vi "Dialog Box.vi"(8 "error in (no error)":errorcluster, 11 "Image Gallery in":refnum<class "Image Gallery.lvclass">) -> (0 "error out":errorcluster, 1 "timed out?":bool, 2 "Selection":string, 3 "Image Gallery out":refnum<class "Image Gallery.lvclass">)   [LabVIEW 2012, in "ImageGallery.lvlib" / "Image Gallery.lvclass"]
doc: "This VI contains the code for the dialog box.\nOverride this VI to provide more functionality or to create your own application-specific dialog box."
uses:
  Image Gallery.lvclass
  Fading/_Fade In(I32).vi
  Fading/_Fade Out(I32).vi
panel:
  in  "Close":bool
  in  "Right":bool
  in  "Left":bool
  out "Picture":picture caption="Caption"
  out "String":string
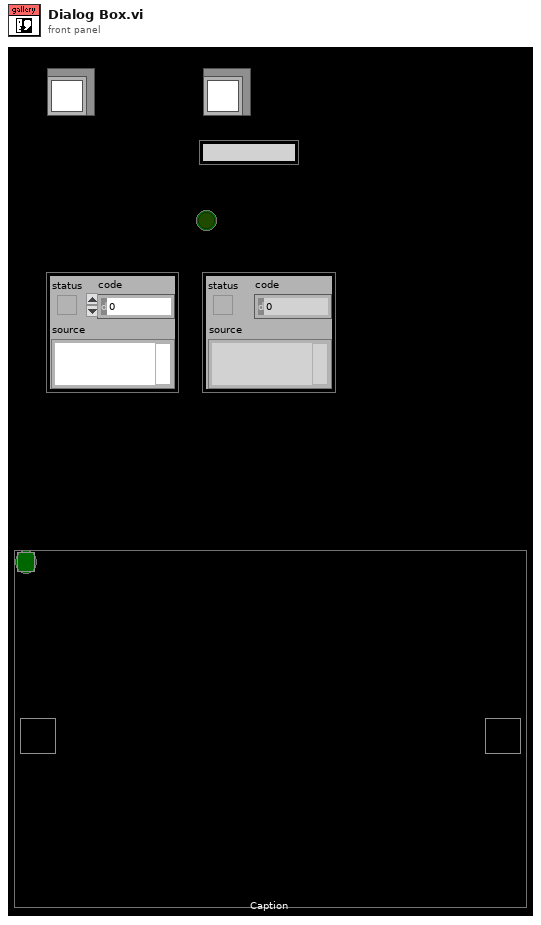
[diagram p1: front panel]
types:
  T1 = cluster{"left":i16, "top":i16, "right":i16, "bottom":i16}
  T2 = typedef "LVPoint32TypeDef.ctl" = cluster{"Horizontal":i32, "Vertical":i32}
  T3 = typedef "LVRectTypeDef.ctl" = cluster{"Left":i16, "Top":i16, "Right":i16, "Bottom":i16}
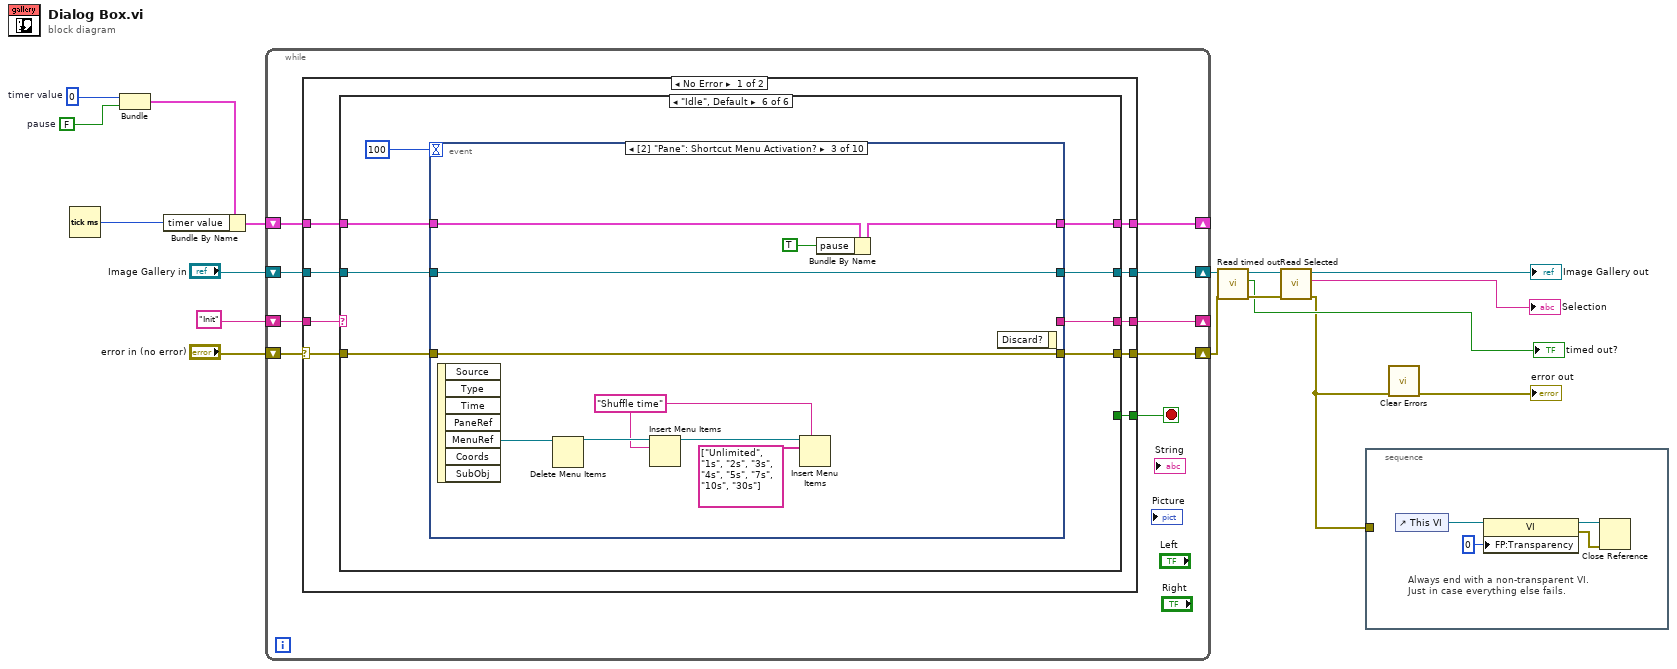
[diagram p0: block diagram]
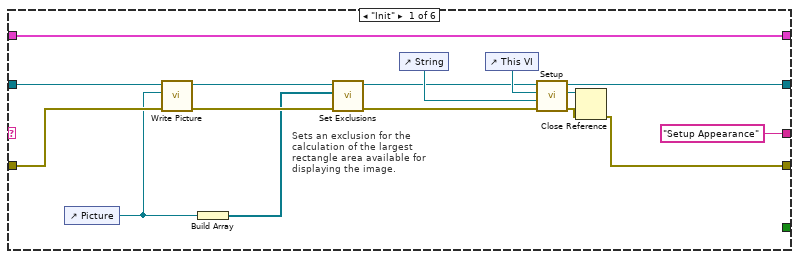
[diagram p2: hidden frame]
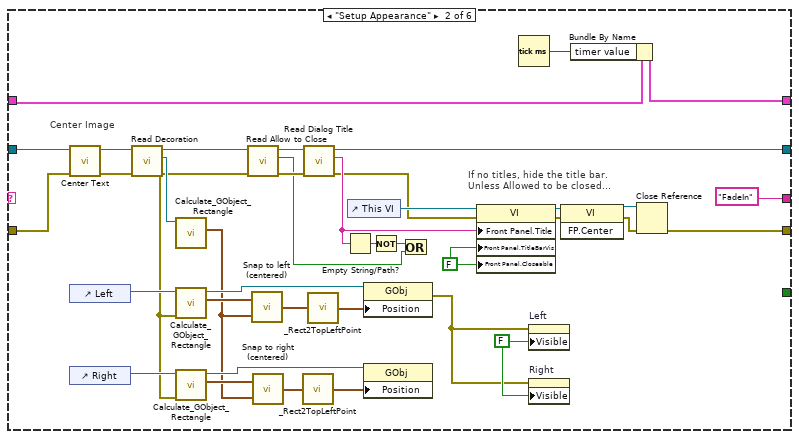
[diagram p3: hidden frame]
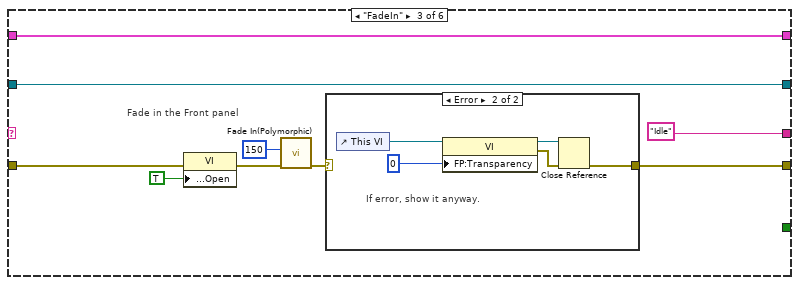
[diagram p4: hidden frame]
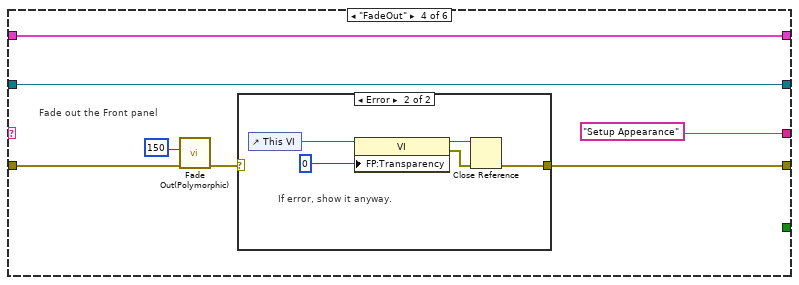
[diagram p6: hidden frame]
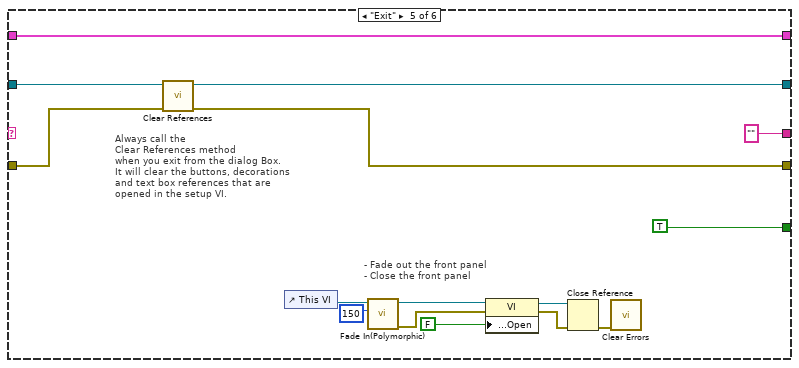
[diagram p8: hidden frame]
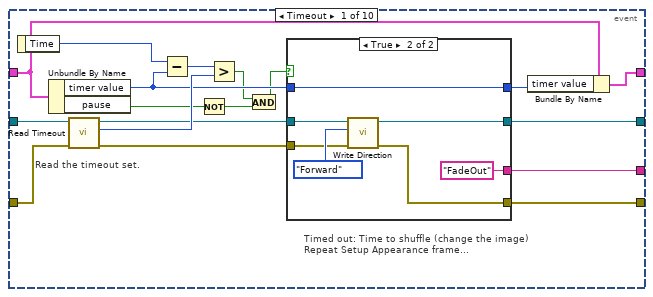
[diagram p9: hidden frame]
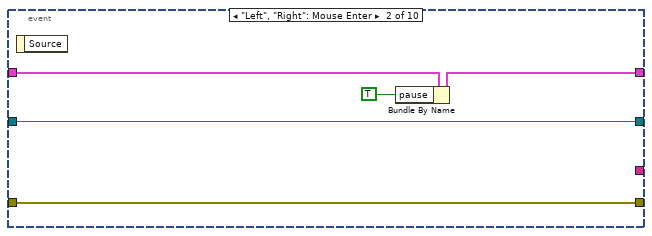
[diagram p11: hidden frame]
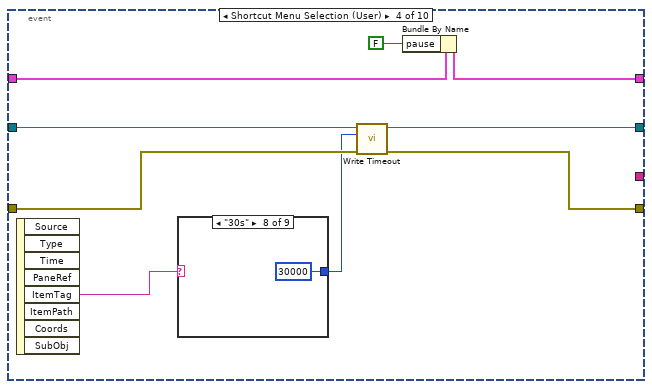
[diagram p12: hidden frame]
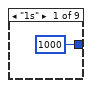
[diagram p13: hidden frame]
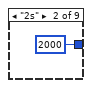
[diagram p14: hidden frame]
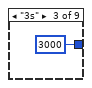
[diagram p15: hidden frame]
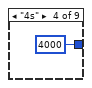
[diagram p16: hidden frame]
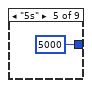
[diagram p17: hidden frame]
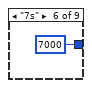
[diagram p18: hidden frame]
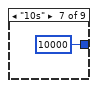
[diagram p19: hidden frame]
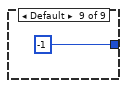
[diagram p20: hidden frame]
diagram:
  w4 = FALSE  # pause
  w5 = u32 0  # timer value
  n1 = Tick Count (ms)() -> (millisecond timer value=w2:u32)
  n2 = Bundle("timer value"=w5, "pause"=w4) -> (w3:cluster{"timer value":u32, "pause":bool})  [unwired: 1 out]
  n3 = Bundle By Name(cluster=w3, "timer value"=w2) -> (w1:cluster{"timer value":u32, "pause":bool})
  n4 = while {
    shift-right: [w22] -> _
    shift-left: "Init" -> [w23]
    shift-right: [w26] -> w16
    shift-left: "Image Gallery in" -> [w25]
    shift-right: [w24] -> w15
    shift-left: "error in (no error)" -> [w20]
    shift-right: [w19] -> _
    shift-left: w1 -> [w18]
    stop <- w21 stop-if-true
    n5 = case shown="No Error" w20 {
      selector: w20 -> [w29 _]
      tunnel: [w35 w250] -> w26
      tunnel: w25 -> [w34 w250]
      tunnel: [w33 errorcluster {"status"=FALSE, "code"=0, "source"=""} ("error out")] -> w24
      tunnel: w23 -> [w32 _]
      tunnel: [w31 "Exit"] -> w22
      tunnel: [w30 _] -> w21
      tunnel: [w28 w247] -> w19
      tunnel: w18 -> [w27 w247]
      frame No Error {
        n6 = case shown="\"Idle\", Default" w32 {
          tunnel: [w49 w81 w99 w112 w123 w141] -> w35
          tunnel: w34 -> [w44 w79 w99 w112 w124 w137]
          tunnel: [w46 w82 w95 w110 w120 w140] -> w33
          tunnel: w29 -> [w43 w78 w94 w107 w122 w136]
          tunnel: ["Setup Appearance" "FadeIn" "Idle" "Setup Appearance" "" w139] -> w31
          tunnel: [_ _ _ _ TRUE _] -> w30
          tunnel: [w36 w52 w91 w106 w119 w134] -> w28
          tunnel: w27 -> [w36 w53 w91 w106 w119 w135]
          frame "Init" {
            # "Sets an exclusion for the\ncalculation of the largest\nrectangle area available for\ndisplaying the image."
            n7 = control-ref of="Picture"() -> (w38:refnum<vi>)
            n8 = call-dynamic "Write Picture.vi"("error in (no error)"=w43, "Picture"=w38, "Image Gallery.lvclass in"=w44) -> ("error out"=w41:errorcluster, "Image Gallery.lvclass out"=w42:refnum<class "Image Gallery.lvclass">)  [unwired: 7 out]
            n9 = Build Array(w38) -> (w37:refnum<vi>[])
            n10 = call-dynamic "Set Exclusions.vi"("error in (no error)"=w41, "Exclusions"=w37, "Dialog in"=w42) -> ("error out"=w39:errorcluster, "Dialog out"=w40:refnum<class "Image Gallery.lvclass">)  [unwired: 7 out]
            n11 = control-ref of="String"() -> (w45:refnum<vi>)
            n12 = control-ref of="This VI"() -> (w50:refnum<vi>)
            n13 = call-dynamic "Setup.vi"("error in (no error)"=w39, "Str Refnum"=w45, "VI Reference"=w50, "Dialog in"=w40) -> ("error out"=w47:errorcluster, "VI reference (dup)"=w48:refnum<vi>, "Dialog out"=w49:refnum<class "Image Gallery.lvclass">)  [unwired: 5 out]
            n14 = Close Reference(reference=w48, error in (no error)=w47) -> (error out=w46:errorcluster)
          }
          frame "Setup Appearance" {
            w56 = FALSE ("Visible")
            w65 = FALSE ("Front Panel Window:Closeable")
            # "Center Image"
            # "If no titles, hide the title bar.\nUnless Allowed to be closed..."
            n15 = call-dynamic "Center Text.vi"("error in (no error)"=w78, "Image Gallery in"=w79) -> ("error out"=w71:errorcluster, "Image Gallery out"=w73:refnum<class "Image Gallery.lvclass">)  [unwired: 8 out]
            n16 = control-ref of="Left"() -> (w69:refnum<vi>)
            n17 = control-ref of="Right"() -> (w66:refnum<vi>)
            n18 = call-dynamic "Read Decoration.vi"("error in (no error)"=w71, "Dialog.lvclass in"=w73) -> ("error out"=w58:errorcluster, "Decoration"=w70:refnum<vi>, "Dialog.lvclass out"=w72:refnum<class "Image Gallery.lvclass">)  [unwired: 7 out]
            n19 = call "Calculate_GObject_Rectangle.vi"("GObject ref"=w70) -> ("Rectangle"=w57:T1)  [unwired: 1 in, 9 out]
            n20 = call "Calculate_GObject_Rectangle.vi"("error in"=w58, "GObject ref"=w69) -> ("Rectangle"=w68:T1, "GObject ref dup"=w62:refnum<vi>)  [unwired: 8 out]
            n21 = call "Calculate_GObject_Rectangle.vi"("error in"=w58, "GObject ref"=w66) -> ("Rectangle"=w67:T1, "GObject ref dup"=w59:refnum<vi>)  [unwired: 8 out]
            n22 = call-dynamic "Read Allow to Close.vi"("error in (no error)"=w58, "Dialog.lvclass in"=w72) -> ("error out"=w76:errorcluster, "Allow to close?"=w74:bool, "Dialog.lvclass out"=w77:refnum<class "Image Gallery.lvclass">)  [unwired: 7 out]
            n23 = call "Snap to left (centered).vi"("Large Rect"=w57, "Small Rect"=w68) -> ("Snapped to left center"=w64:T1)
            n24 = call "Snap to right (centered).vi"("Large Rect"=w57, "Small Rect"=w67) -> ("Snapped to right center"=w60:T1)
            n25 = call "_Rect2TopLeftPoint.vi"("bounds"=w60) -> ("TopLeft point"=w61:cluster{"x":i32, "y":i32})  [unwired: 4 out]
            n26 = call-dynamic "Read Dialog Title.vi"("error in (no error)"=w76, "Dialog in"=w77) -> ("error out"=w80:errorcluster, "Dialog Title"=w85:string, "Dialog out"=w81:refnum<class "Image Gallery.lvclass">)  [unwired: 7 out]
            n27 = call "_Rect2TopLeftPoint.vi"("bounds"=w64) -> ("TopLeft point"=w63:cluster{"x":i32, "y":i32})  [unwired: 4 out]
            n28 = Empty String/Path?(string/path=w85) -> (empty?=w88:bool)
            n29 = control-ref of="This VI"() -> (w89:refnum<vi>)
            n30 = property class="GObj"(reference=w62, "Position"=w63) -> (error out=w55:errorcluster)  [unwired: 1 in, 1 out]
            n31 = property class="GObj"(reference=w59, "Position"=w61) -> ()  [unwired: 1 in, 2 out]
            n32 = Not(x=w88) -> (.not. x?=w75:bool)
            n33 = Or(x=w75, y=w74) -> ()  [unwired: 1 out]
            n34 = property class="VI"(reference=w89, error in=w80, "Front Panel.Title"=w85, "Front Panel.TitleBarVis"=w65, "Front Panel.Closeable"=w65) -> (reference out=w87:refnum<vi>, error out=w86:errorcluster)
            n35 = Tick Count (ms)() -> (millisecond timer value=w54:u32)
            n36 = property on="Left" class="Bool"(error in=w55, "Visible"=w56) -> ()  [unwired: 1 in, 2 out]
            n37 = property on="Right" class="Bool"(error in=w55, "Visible"=w56) -> ()  [unwired: 1 in, 2 out]
            n38 = invoke class="VI" method="FP.Center"(reference=w87, error in=w86) -> (reference out=w84:refnum<vi>, error out=w83:errorcluster)  [unwired: 1 in, 1 out]
            n39 = Bundle By Name(cluster=w53, "timer value"=w54) -> (w52:cluster{"timer value":u32, "pause":bool})
            n40 = Close Reference(reference=w84, error in (no error)=w83) -> (error out=w82:errorcluster)
          }
          frame "FadeIn" {
            # "Fade in the Front panel"
            n41 = property class="VI"(error in=w94, "Front Panel.Open"=TRUE ("Front Panel Window:Open")) -> (error out=w93:errorcluster)  [unwired: 1 in, 1 out]
            n42 = call-poly "Fade In(Polymorphic).vi"("error in"=w93, "Fade time (ms)"=150) -> ("error out"=w96:errorcluster)  [unwired: 2 in, 7 out]
            n43 = case shown="Error" w96 {
              selector: w96 -> [w100 _]
              tunnel: [w100 w101] -> w95
              frame No Error {
              }
              frame Error {
                # "If error, show it anyway."
                n44 = control-ref of="This VI"() -> (w103:refnum<vi>)
                n45 = property class="VI"(reference=w103, "FP:Transparency"=u8 0 ("Front Panel Window:Transparency")) -> (reference out=w104:refnum<vi>, error out=w105:errorcluster)  [unwired: 1 in]
                n46 = Close Reference(reference=w104, error in (no error)=w105) -> (error out=w101:errorcluster)
              }
            }
          }
          frame "FadeOut" {
            # "Fade out the Front panel"
            n47 = call-poly "Fade Out(Polymorphic).vi"("error in"=w107, "Fade time (ms)"=150) -> ("error out"=w108:errorcluster)  [unwired: 2 in, 7 out]
            n48 = case shown="Error" w108 {
              selector: w108 -> [w113 _]
              tunnel: [w113 w114] -> w110
              frame No Error {
              }
              frame Error {
                # "If error, show it anyway."
                n49 = control-ref of="This VI"() -> (w116:refnum<vi>)
                n50 = property class="VI"(reference=w116, "FP:Transparency"=u8 0 ("Front Panel Window:Transparency")) -> (reference out=w117:refnum<vi>, error out=w118:errorcluster)  [unwired: 1 in]
                n51 = Close Reference(reference=w117, error in (no error)=w118) -> (error out=w114:errorcluster)
              }
            }
          }
          frame "Exit" {
            # "Always call the\nClear References method\nwhen you exit from the dialog Box.\nIt will clear the buttons, decorations\nand text box references that are \nopened in the setup VI."
            # "- Fade out the front panel\n- Close the front panel"
            n52 = call-dynamic "Clear References.vi"("error in (no error)"=w122, "Dialog in"=w124) -> ("error out"=w120:errorcluster, "Dialog out"=w123:refnum<class "Image Gallery.lvclass">)  [unwired: 8 out]
            n53 = control-ref of="This VI"() -> (w130:refnum<vi>)
            n54 = call-poly "Fade In(Polymorphic).vi"("Fade time (ms)"=150, "VI Reference (calling VI)"=w130) -> ("error out"=w128:errorcluster, "dup VI Reference"=w129:refnum<vi>)  [unwired: 2 in, 6 out]
            n55 = property class="VI"(reference=w129, error in=w128, "Front Panel.Open"=FALSE ("Front Panel Window:Open")) -> (reference out=w126:refnum<vi>, error out=w125:errorcluster)
            n56 = Close Reference(reference=w126, error in (no error)=w125) -> (error out=w121:errorcluster)
            n57 = call <vilib>:"Clear Errors.vi"("error in (no error)"=w121) -> ()  [unwired: 7 out]
          }
          frame "Idle", Default {
            n58 = event shown="[2] \"Pane\": Shortcut Menu Activation?" {
              selector: _ -> [_ _ _ _ _ _ _ _ _ _]
              dyn-events: _ -> [_ _ _ _ _ _ _ _ _ _]
              timeout: 100 -> [_ _ _ _ _ _ _ _ _ _]
              tunnel: [w158 w171 w181 w189 w204 w217 w224 w233 w240 w245] -> w141
              tunnel: w137 -> [w152 w171 w181 w190 w204 w217 w227 w236 w240 w245]
              tunnel: [w157 w170 w180 w187 w203 w216 w223 w232 w239 w244] -> w140
              tunnel: w136 -> [w155 w170 w180 w188 w203 w216 w226 w235 w239 w244]
              tunnel: [w159 _ _ _ _ _ "FadeOut" "FadeOut" "Exit" "Exit"] -> w139
              tunnel: w135 -> [w146 w174 w184 w193 w207 w219 w221 w230 w238 w243]
              tunnel: [w147 w173 w183 w192 w206 w219 w220 w229 w238 w243] -> w134
              event Timeout {
                # "Read the timeout set."
                # "Timed out: Time to shuffle (change the image)\nRepeat Setup Appearance frame..."
                n59 = event-data() -> ("Time"=w150:u32)  [unwired: 1 out]
                n60 = Unbundle By Name(w146) -> ("timer value"=w149:u32, "pause"=w145:bool)
                n61 = call-dynamic "Read Timeout.vi"("error in (no error)"=w155, "Dialog.lvclass in"=w152) -> ("error out"=w153:errorcluster, "Timeout"=w154:i32, "Dialog.lvclass out"=w151:refnum<class "Image Gallery.lvclass">)  [unwired: 7 out]
                n62 = Subtract(x=w150, y=w149) -> (x-y=w156:u32)
                n63 = Not(x=w145) -> (.not. x?=w144:bool)
                n64 = Greater?(x=w156, y=w154) -> (0:w143:bool)
                n65 = And(x=w143, y=w144) -> (x .and. y?=w142:bool)
                n66 = case shown="True" w142 {
                  tunnel: [_ "FadeOut"] -> w159
                  tunnel: [w162 w167] -> w158
                  tunnel: [w161 w166] -> w157
                  tunnel: w151 -> [w162 w165]
                  tunnel: w153 -> [w161 w164]
                  tunnel: w149 -> [w160 w163]
                  tunnel: [w160 w163] -> w148
                  frame False {
                  }
                  frame True {
                    n67 = call-dynamic "Write Direction.vi"("error in (no error)"=w164, "Direction"=enum16{"Forward", "Backward"}."Forward", "Image Gallery.lvclass in"=w165) -> ("error out"=w166:errorcluster, "Image Gallery.lvclass out"=w167:refnum<class "Image Gallery.lvclass">)  [unwired: 7 out]
                  }
                }
                n68 = Bundle By Name(cluster=w146, "timer value"=w148) -> (w147:cluster{"timer value":u32, "pause":bool})
              }
              event "Left", "Right": Mouse Enter {
                n69 = event-data() -> ()  [unwired: 2 out]
                n70 = Bundle By Name(cluster=w174, "pause"=TRUE) -> (w173:cluster{"timer value":u32, "pause":bool})
              }
              event Shortcut Menu Activation? {
                w177 = "Shuffle time"
                n71 = event-data() -> ("MenuRef"=w179:refnum<k9>)  [unwired: 7 out]
                n72 = Delete Menu Items(9:w179) -> (3:w178:refnum<k9>)  [unwired: 1 in, 3 out]
                n73 = Insert Menu Items(8:w177, 9:w178) -> (3:w176:refnum<k9>)  [unwired: 1 in, 5 out]
                n74 = Insert Menu Items(5:w177, 8:string[] ["Unlimited", "1s", "2s", "3s", "4s", "5s", "7s", "10s", "30s"] ("item names"), 9:w176) -> ()  [unwired: 1 in, 5 out]
                n75 = Bundle By Name(cluster=w184, "pause"=TRUE) -> (w183:cluster{"timer value":u32, "pause":bool})
                n76 = event-data() -> ()  [unwired: 1 in, 2 out]
              }
              event Shortcut Menu Selection (User) {
                n77 = event-data() -> ("ItemTag"=w186:string)  [unwired: 8 out]
                n78 = case shown="\"30s\"" w186 {
                  tunnel: [1000 ("Timeout") 2000 ("Timeout") 3000 ("Timeout") 4000 ("Timeout") 5000 ("Timeout") 7000 ("Timeout") 10000 ("Timeout") 30000 ("Timeout") -1 ("Timeout")] -> w185
                  frame "1s" {
                  }
                  frame "2s" {
                  }
                  frame "3s" {
                  }
                  frame "4s" {
                  }
                  frame "5s" {
                  }
                  frame "7s" {
                  }
                  frame "10s" {
                  }
                  frame "30s" {
                  }
                  frame Default {
                  }
                }
                n79 = call-dynamic "Write Timeout.vi"("error in (no error)"=w188, "Timeout"=w185, "Dialog.lvclass in"=w190) -> ("error out"=w187:errorcluster, "Dialog.lvclass out"=w189:refnum<class "Image Gallery.lvclass">)  [unwired: 7 out]
                n80 = Bundle By Name(cluster=w193, "pause"=FALSE) -> (w192:cluster{"timer value":u32, "pause":bool})
              }
              event "Left", "Right": Mouse Leave {
                n81 = event-data() -> ()  [unwired: 2 out]
                n82 = Bundle By Name(cluster=w207, "pause"=FALSE) -> (w206:cluster{"timer value":u32, "pause":bool})
              }
              event Mouse Move {
                n83 = event-data() -> ("Coords"=w210:T2)  [unwired: 2 out]
                n84 = property class="VI"() -> ("Front Panel.PanelBounds"=w208:T3)  [unwired: 2 in, 2 out]
                n85 = call "WindowsBoundsToRect.vi"("Windows Bounds"=w208) -> ("Rectangle"=w209:T1)  [unwired: 10 out]
                n86 = call "Divide Rectangle.vi"("Band (50)"=i16 50, "Coords"=w210, "Rectangle"=w209) -> ("Zone"=w212:i32)  [unwired: 8 out]
                n87 = Equal?(x=4, y=w212) -> (x = y?=w214:bool)
                n88 = Equal?(x=5, y=w212) -> (x = y?=w211:bool)
                n89 = property on="Left" class="Bool"("Visible"=w214) -> ()  [unwired: 2 in, 2 out]
                n90 = property on="Right" class="Bool"("Visible"=w211) -> ()  [unwired: 2 in, 2 out]
              }
              event "Left": Value Change {
                # "Timed out: Time to shuffle (change the image)\nRepeat Setup Appearance frame..."
                n91 = event-data() -> ()  [unwired: 7 out]
                n92 = call-dynamic "Write Direction.vi"("error in (no error)"=w226, "Direction"=enum16{"Forward", "Backward"}."Backward", "Image Gallery.lvclass in"=w227) -> ("error out"=w223:errorcluster, "Image Gallery.lvclass out"=w224:refnum<class "Image Gallery.lvclass">)  [unwired: 7 out]
                n93 = Tick Count (ms)() -> (millisecond timer value=w222:u32)
                n94 = Bundle By Name(cluster=w221, "timer value"=w222) -> (w220:cluster{"timer value":u32, "pause":bool})
              }
              event "Right": Value Change {
                # "Timed out: Time to shuffle (change the image)\nRepeat Setup Appearance frame..."
                n95 = event-data() -> ()  [unwired: 7 out]
                n96 = call-dynamic "Write Direction.vi"("error in (no error)"=w235, "Direction"=enum16{"Forward", "Backward"}."Forward", "Image Gallery.lvclass in"=w236) -> ("error out"=w232:errorcluster, "Image Gallery.lvclass out"=w233:refnum<class "Image Gallery.lvclass">)  [unwired: 7 out]
                n97 = Tick Count (ms)() -> (millisecond timer value=w231:u32)
                n98 = Bundle By Name(cluster=w230, "timer value"=w231) -> (w229:cluster{"timer value":u32, "pause":bool})
              }
              event Panel Close? {
                # "Panel closed by user."
                n99 = event-data() -> ()  [unwired: 4 out]
                n100 = event-data("Discard?"=TRUE) -> ()  [unwired: 1 in, 1 out]
              }
              event "Close": Value Change {
                # "Panel closed by user."
                n101 = event-data() -> ()  [unwired: 7 out]
              }
            }
          }
        }
      }
      frame Error {
        # "Report the error in the log if necessary..."
      }
    }
  }
  n102 = call-dynamic "Read timed out.vi"("error in (no error)"=w15, "Dialog.lvclass in"=w16) -> ("error out"=w13:errorcluster, "timed out?"=→"timed out?":bool, "Dialog.lvclass out"=w14:refnum<class "Image Gallery.lvclass">)  [unwired: 7 out]
  n103 = call-dynamic "Read Selected.vi"("error in (no error)"=w13, "Dialog.lvclass in"=w14) -> ("error out"=w7:errorcluster, "Selected"=→"Selection":string, "Dialog.lvclass out"=→"Image Gallery out":refnum<class "Image Gallery.lvclass">)  [unwired: 7 out]
  n104 = stacked-sequence {
    tunnel: w7 -> [_]
    frame #0 {
      # "Always end with a non-transparent VI.\nJust in case everything else fails."
      n105 = control-ref of="This VI"() -> (w253:refnum<vi>)
      n106 = property class="VI"(reference=w253, "FP:Transparency"=u8 0 ("Front Panel Window:Transparency")) -> (reference out=w252:refnum<vi>, error out=w251:errorcluster)  [unwired: 1 in]
      n107 = Close Reference(reference=w252, error in (no error)=w251) -> ()  [unwired: 1 out]
    }
  }
  n108 = call <vilib>:"Clear Errors.vi"("error in (no error)"=w7) -> ("error out"=→"error out":errorcluster)  [unwired: 6 out]
